vi "KeyenceCVX.GetImagePaths.vi"(8 "error in":errorcluster, 10 "ImageFolder":path, 11 "FTPPath":path) -> (0 "error out":errorcluster, 2 "ImgPathB":path, 3 "ImgPathA":path)   [LabVIEW 2016]
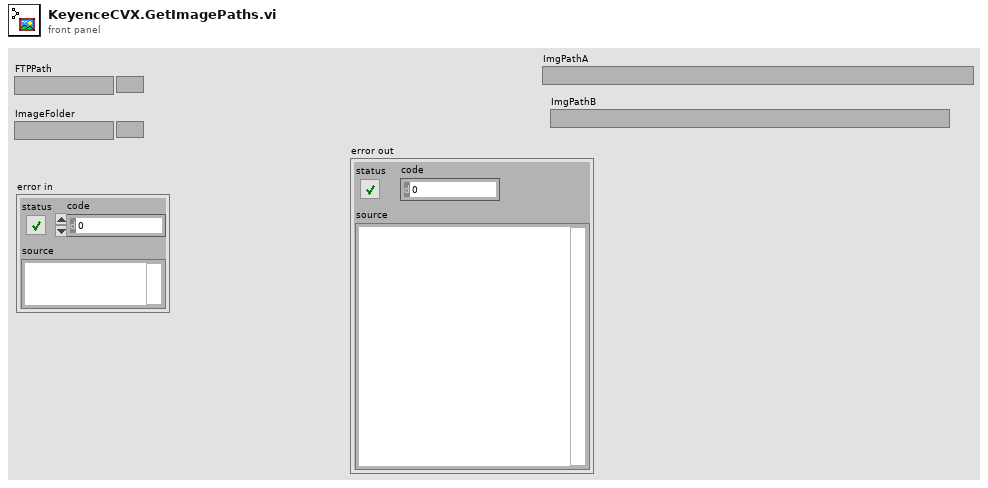
[diagram p1: front panel]
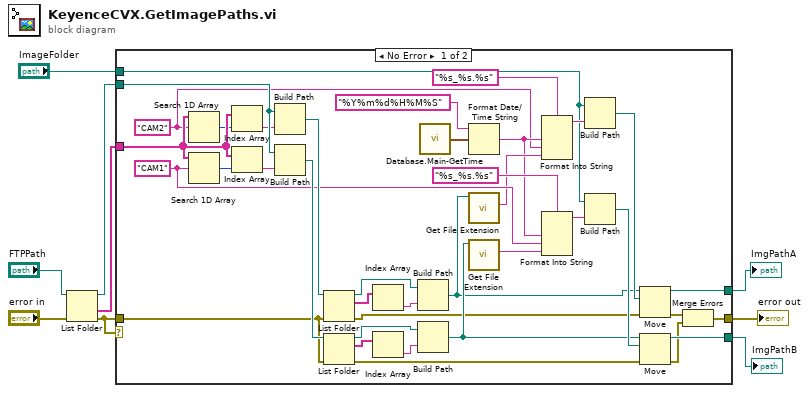
[diagram p0: block diagram]
diagram:
  n1 = List Folder(path="FTPPath", error in="error in") -> (path out=w9:path, folder names=w8:string[], error out=w2:errorcluster)  [unwired: 2 in, 1 out]
  n2 = case shown="No Error" w2 {
    tunnel: w9 -> [w38 _]
    tunnel: w8 -> [w36 _]
    tunnel: w2 -> [w33 w48]
    tunnel: [w15 _] -> w5
    tunnel: [w14 _] -> w4
    tunnel: [w11 w48] -> w3
    tunnel: "ImageFolder" -> [w10 _]
    frame No Error {
      w29 = "CAM1" ("element")
      w24 = "CAM2" ("element")
      n3 = Search 1D Array(1D array=w36, element=w24) -> (index of element=w34:i32)  [unwired: 1 in]
      n4 = Search 1D Array(1D array=w36, element=w29) -> (index of element=w35:i32)  [unwired: 1 in]
      n5 = Index Array(array=w36, index=w34) -> (element=w37:string)
      n6 = Index Array(array=w36, index=w35) -> (element=w39:string)
      n7 = Build Path(base path=w38, name or relative path=w37) -> (appended path=w40:path)
      n8 = Build Path(base path=w38, name or relative path=w39) -> (appended path=w41:path)
      n9 = List Folder(path=w40, error in=w33) -> (path out=w42:path, filenames=w43:string[], error out=w17:errorcluster)  [unwired: 2 in, 1 out]
      n10 = List Folder(path=w41, error in=w33) -> (path out=w46:path, filenames=w47:string[], error out=w16:errorcluster)  [unwired: 2 in, 1 out]
      n11 = Index Array(array=w43) -> (element=w44:string)  [unwired: 1 in]
      n12 = Index Array(array=w47) -> (element=w45:string)  [unwired: 1 in]
      n13 = Build Path(base path=w42, name or relative path=w44) -> (appended path=w18:path)
      n14 = Build Path(base path=w46, name or relative path=w45) -> (appended path=w21:path)
      n15 = call "Database.Main-GetTime.vi"() -> ("TS"=w31:timestamp)  [unwired: 1 in]
      n16 = Format Date/Time String(time format string (%c)="%Y%m%d%H%M%S", seconds (now)=w31) -> (date/time string=w25:string)  [unwired: 1 in]
      n17 = call <vilib>:"Get File Extension.vi"("file"=w18) -> ("lowercase file extension"=w27:string)  [unwired: 6 in, 4 out]
      n18 = call <vilib>:"Get File Extension.vi"("file"=w21) -> ("lowercase file extension"=w28:string)  [unwired: 6 in, 4 out]
      n19 = Format Into String(format string="%s_%s.%s", w25, w24, w27) -> (resulting string=w19:string)  [unwired: 2 in, 1 out]
      n20 = Format Into String(format string="%s_%s.%s", w25, w29, w28) -> (resulting string=w23:string)  [unwired: 2 in, 1 out]
      n21 = Build Path(base path=w10, name or relative path=w19) -> (appended path=w20:path)
      n22 = Build Path(base path=w10, name or relative path=w23) -> (appended path=w22:path)
      n23 = Move(source path=w18, error in=w17, 10:w20) -> (error out=w13:errorcluster, 3:w14:path)  [unwired: 2 in, 1 out]
      n24 = Move(source path=w21, error in=w16, 10:w22) -> (error out=w12:errorcluster, 3:w15:path)  [unwired: 2 in, 1 out]
      n25 = Merge Errors(w13, w12) -> (w11:errorcluster)
    }
    frame Error {
    }
  }
  "error out" <- w3
  "ImgPathB" <- w5
  "ImgPathA" <- w4
